vi "Delete from Object.vi"(5 "Item Name":string, 6 "Object (or Item) Path":string, 7 "error in (no error)":errorcluster, 9 "Object Offset":i32, 10 "JSON in":string="{}") -> (0 "error out":errorcluster, 1 "<JSON>Deleted":string, 2 "Found and Deleted":bool, 3 "<JSON>":string)   [LabVIEW 2015, in "JSONtext.lvlib"]
doc: "Deleates JSON item at the Path specified."
uses:
  JSONtext.lvlib
  Parsing State.ctl
  support/quote and escape json string 2.vi
  Advance past whitespace.vi
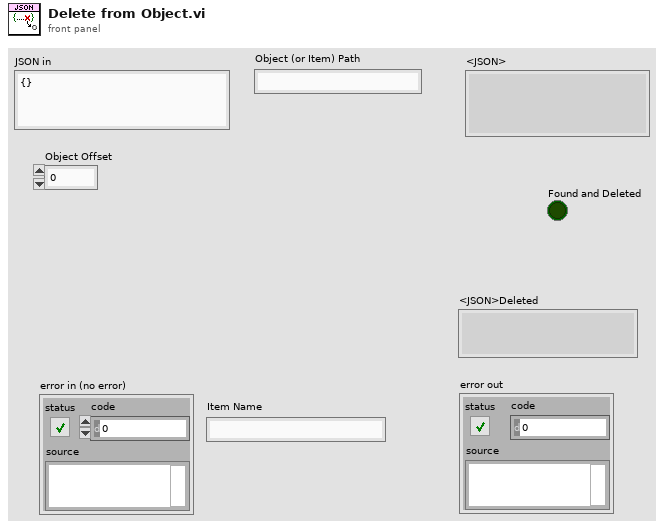
[diagram p1: front panel]
types:
  T1 = typedef "JSONtext.lvlib/Parsing State.ctl" = enum16{"Parser Error", "Object", "Array", "String", "Number/Other", "Leading Whitespace", "Object end", "Array end", "Value end"}
  T2 = typedef "JSONtext.lvlib/Found Items.ctl" = cluster{"Item offset":i32, "Offset past Item":i32, "Name offset":i32, "Offset past Name":i32, "Found":bool, "Item Type":T1, "Item Index":i32}
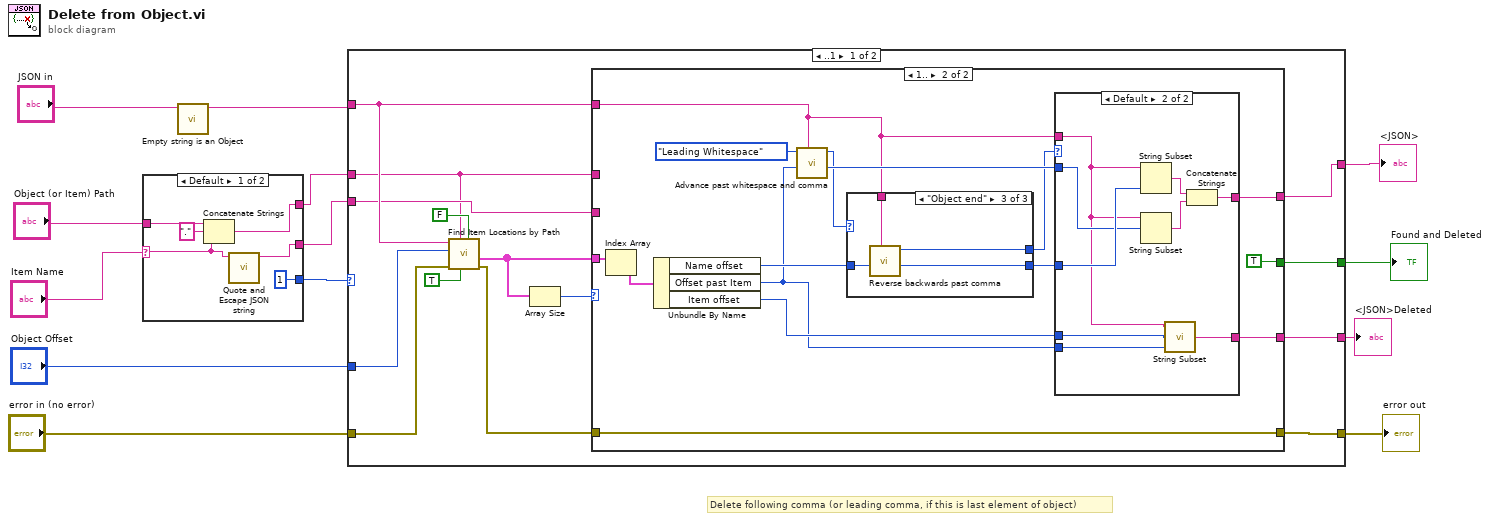
[diagram p0: block diagram]
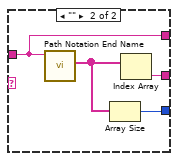
[diagram p2: hidden frame]
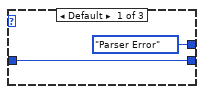
[diagram p4: hidden frame]
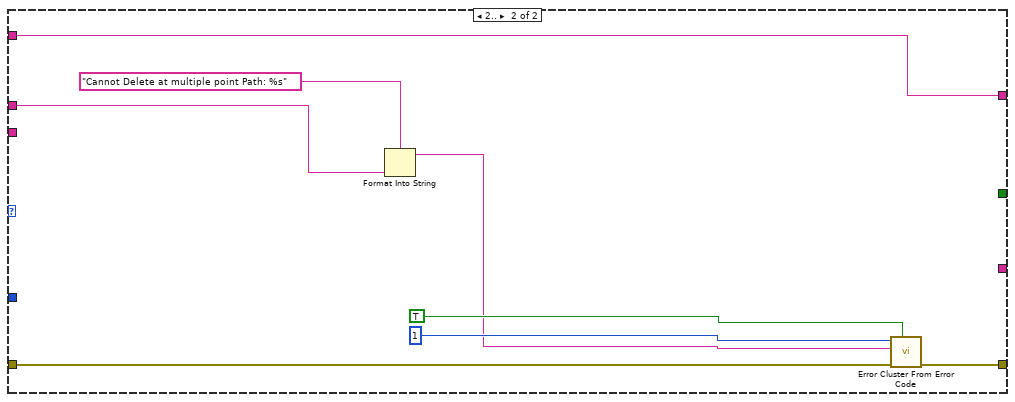
[diagram p7: hidden frame]
diagram:
  # "Delete following comma (or leading comma, if this is last element of object)"
  n1 = case shown="Default" "Item Name" {
    selector: "Item Name" -> [w15 _]
    tunnel: [w14 w23] -> w8
    tunnel: [1 w22] -> w7
    tunnel: "Object (or Item) Path" -> [w19 w20]
    tunnel: [w17 w20] -> w4
    frame Default {
      n2 = Concatenate Strings(w19, "." ("string"), w15) -> (w17:string)
      n3 = call "Quote and Escape JSON string.vi"("Plain Text"=w15) -> ("<JSON>"=w14:string)  [unwired: 10 in]
    }
    frame "" {
      n4 = call "Path Notation End Name.vi"("Item Path"=w20) -> ("<JSON>End Names"=w21:string[])  [unwired: 10 in]
      n5 = Array Size(array=w21) -> (size(s)=w22:i32)
      n6 = Index Array(array=w21) -> (element=w23:string)  [unwired: 1 in]
    }
  }
  n7 = call "Empty string is an Object.vi"("JSON Input"="JSON in") -> ("<JSON>Object"=w2:string)  [unwired: 10 in]
  n8 = case shown="..1" w7 {
    tunnel: [w37 w74] -> w13
    tunnel: w2 -> [w36 w74]
    tunnel: "Object Offset" -> [w35 _]
    tunnel: [w33 _] -> w11
    tunnel: "error in (no error)" -> [w32 w75]
    tunnel: [w25 w78] -> w9
    tunnel: w8 -> [w30 _]
    tunnel: w4 -> [w27 w73]
    tunnel: [w24 _] -> w1
    frame ..1 {
      n9 = call "Find Item Locations by Path.vi"("Insertion point if not found"=FALSE, "Only return first found"=TRUE, "Path"=w27, "error in (no error)"=w32, "Object Offset"=w35, "JSON"=w36) -> ("error out"=w26:errorcluster, "Items"=w29:T2[])  [unwired: 4 in]
      n10 = Array Size(array=w29) -> (size(s)=w28:i32)
      n11 = case shown="1.." w28 {
        tunnel: [w39 w49] -> w37
        tunnel: w36 -> [w39 w46]
        tunnel: w29 -> [_ w54]
        tunnel: [_ TRUE] -> w33
        tunnel: w30 -> [_ _]
        tunnel: w26 -> [w38 w53]
        tunnel: w27 -> [_ _]
        tunnel: [w38 w53] -> w25
        tunnel: [_ w40] -> w24
        frame 0, Default {
        }
        frame 1.. {
          n12 = Index Array(array=w54) -> (element=w51:T2)  [unwired: 1 in]
          n13 = Unbundle By Name(w51) -> ("Name offset"=w48:i32, "Offset past Item"=w41:i32, "Item offset"=w42:i32)
          n14 = call "Advance past whitespace and comma.vi"("JSON"=w46, "Offset"=w41, "State in"=Parsing_State."Leading Whitespace") -> ("Offset past match"=w50:i32, "State"=w45:T1)  [unwired: 7 in]
          n15 = case shown="\"Object end\"" w45 {
            selector: w45 -> [_ w57 _]
            tunnel: w48 -> [w56 w58 w62]
            tunnel: [w56 w58 w61] -> w47
            tunnel: w46 -> [_ _ w60]
            tunnel: [Parsing_State."Parser Error" ("Parser State") w57 w59] -> w44
            frame Default {
            }
            frame "Object".."Number/Other" {
            }
            frame "Object end" {
              n16 = call "Reverse backwards past comma.vi"("JSON"=w60, "Offset"=w62) -> ("Offset of first non-whitespace"=w61:i32, "Parser State"=w59:T1)  [unwired: 8 in]
            }
          }
          n17 = case shown="Default" w44 {
            tunnel: w46 -> [w63 w67]
            tunnel: w47 -> [_ w72]
            tunnel: w50 -> [_ w71]
            tunnel: [w63 w68] -> w49
            tunnel: w42 -> [_ w66]
            tunnel: w41 -> [_ w65]
            tunnel: [_ w64] -> w40
            frame "Parser Error" {
            }
            frame Default {
              n18 = String Subset(string=w67, length (rest)=w72) -> (substring=w70:string)  [unwired: 1 in]
              n19 = String Subset(string=w67, offset (0)=w71) -> (substring=w69:string)  [unwired: 1 in]
              n20 = call "String Subset.vi"("Offset past End"=w65, "Start offset"=w66, "JSON"=w67) -> ("substring"=w64:string)  [unwired: 2 in]
              n21 = Concatenate Strings(w70, w69) -> (w68:string)
            }
          }
        }
      }
    }
    frame 2.. {
      n22 = Format Into String(format string="Cannot Delete at multiple point Path: %s", w73) -> (resulting string=w76:string)  [unwired: 2 in, 1 out]
      n23 = call <vilib>:"Error Cluster From Error Code.vi"("show call chain? (False)"=TRUE, "error in (no error)"=w75, "error message (\"\")"=w76, "error code (0)"=1) -> ("error out"=w78:errorcluster)  [unwired: 5 in]
    }
  }
  "Found and Deleted" <- w11
  "<JSON>" <- w13
  "error out" <- w9
  "<JSON>Deleted" <- w1
